vi "AESC#vi.vi"(7 "枚举":enum16{"AesEncrypt", "AesDecrypt"}(ring), 8 "错误输入（无错误）":errorcluster, 9 "encryptStr":string, 10 "key":string, 11 "plainText":string) -> (0 "错误输出":errorcluster, 2 "AESDecrypt":string, 3 "AESEncrypt":string)   [LabVIEW 2016, in "数据传输系统-05.lvlib"]
uses:
  data/AESTOOL.dll
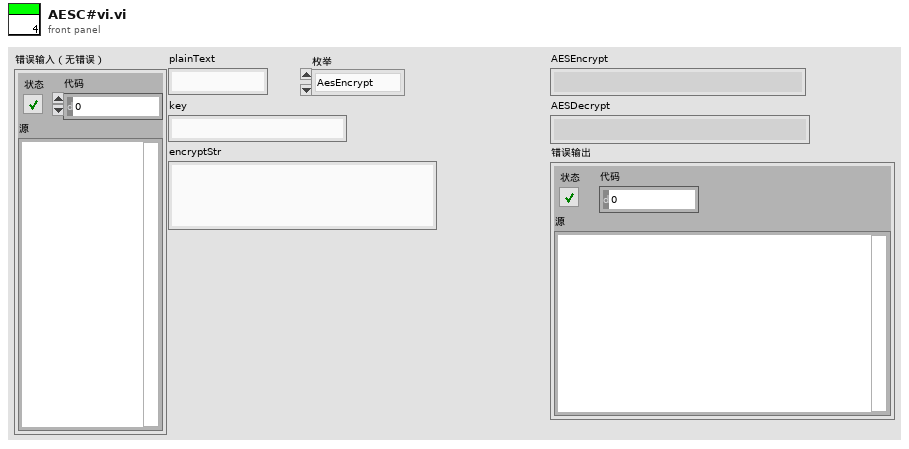
[diagram p1: front panel]
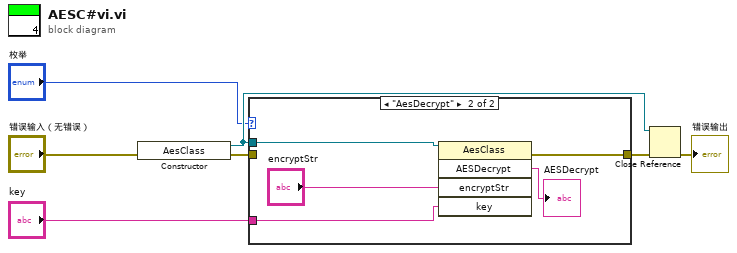
[diagram p0: block diagram]
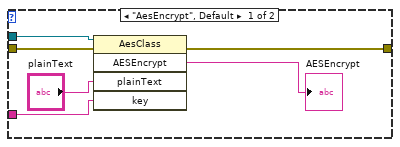
[diagram p2: hidden frame]
diagram:
  n1 = constructor class="AesClass"(error in="错误输入（无错误）") -> (reference out=w4:refnum<k24>, error out=w7:errorcluster)  [unwired: 2 in, 1 out]
  n2 = case shown="\"AesDecrypt\"" "枚举" {
    tunnel: w7 -> [w13 _]
    tunnel: [w10 w14] -> w5
    tunnel: w4 -> [w9 w18]
    tunnel: "key" -> [w8 w16]
    frame "AesEncrypt", Default {
      n3 = invoke class="AesClass" method="AESEncrypt"(reference=w9, error in=w13, "plainText"="plainText", "key"=w8) -> (error out=w10:errorcluster, "AESEncrypt"=→"AESEncrypt":string)  [unwired: 1 in, 3 out]
    }
    frame "AesDecrypt" {
      n4 = invoke on="调用节点" class="AesClass" method="AESDecrypt"(reference=w18, "encryptStr"="encryptStr", "key"=w16) -> (error out=w14:errorcluster, "AESDecrypt"=→"AESDecrypt":string)  [unwired: 2 in, 3 out]
    }
  }
  n5 = Close Reference(reference=w4, error in (no error)=w5) -> (error out=→"错误输出":errorcluster)
